vi "add_Inertia.vi"(6 "Inertia":T1, 7 "msg in":string) -> (3 "msg out":string)   [LabVIEW 2016]
doc: "Flattens an inertia with covariance into a message"
uses:
  std_msgs/subs/float64Scalar.vi
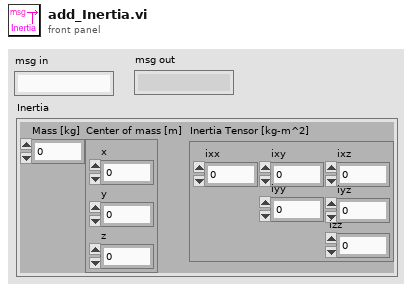
[diagram p1: front panel]
types:
  T1 = cluster{"Mass [kg]":dbl, "Center of mass [m]":cluster{"x":dbl, "y":dbl, "z":dbl}, "Inertia Tensor [kg-m^2]":cluster{"ixx":dbl, "ixy":dbl, "ixz":dbl, "iyy":dbl, "iyz":dbl, "izz":dbl}}
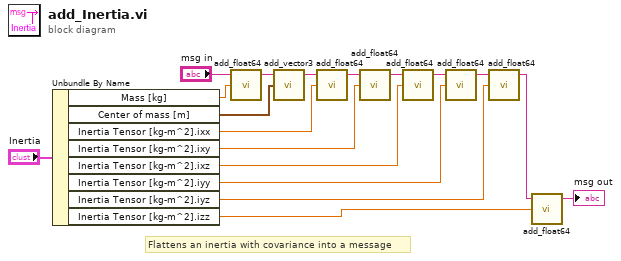
[diagram p0: block diagram]
diagram:
  # "Flattens an inertia with covariance into a message"
  n1 = Unbundle By Name("Inertia") -> ("Mass [kg]"=w1:dbl, "Center of mass [m]"=w2:cluster{"x":dbl, "y":dbl, "z":dbl}, "Inertia Tensor [kg-m^2].ixx"=w13:dbl, "Inertia Tensor [kg-m^2].ixy"=w12:dbl, "Inertia Tensor [kg-m^2].ixz"=w11:dbl, "Inertia Tensor [kg-m^2].iyy"=w10:dbl, "Inertia Tensor [kg-m^2].iyz"=w9:dbl, "Inertia Tensor [kg-m^2].izz"=w8:dbl)
  n2 = call-poly "add_float64.vi"("Numeric"=w1, "msg in"="msg in") -> ("msg out"=w17:string)  [unwired: 3 in]
  n3 = call "add_vector3.vi"("Vector3"=w2, "msg in"=w17) -> ("msg out"=w15:string)  [unwired: 3 in]
  n4 = call-poly "add_float64.vi"("Numeric"=w13, "msg in"=w15) -> ("msg out"=w14:string)  [unwired: 3 in]
  n5 = call-poly "add_float64.vi"("Numeric"=w12, "msg in"=w14) -> ("msg out"=w16:string)  [unwired: 3 in]
  n6 = call-poly "add_float64.vi"("Numeric"=w11, "msg in"=w16) -> ("msg out"=w7:string)  [unwired: 3 in]
  n7 = call-poly "add_float64.vi"("Numeric"=w10, "msg in"=w7) -> ("msg out"=w6:string)  [unwired: 3 in]
  n8 = call-poly "add_float64.vi"("Numeric"=w9, "msg in"=w6) -> ("msg out"=w5:string)  [unwired: 3 in]
  n9 = call-poly "add_float64.vi"("Numeric"=w8, "msg in"=w5) -> ("msg out"=→"msg out":string)  [unwired: 3 in]
